vi "Get Distance LUT.vi"() -> (2 "Info":T1, 3 "LUT Out":i32[](array[numeric])=[0, 3, 6, 9, 12])   [LabVIEW 2025]
panel:
  in  "Outputs":T1
  out "Max Distance":i32
  out "Step Size":i32=3
  out "Start Distance":i32
  in  "Distance LUT":i32[](array[numeric])=[6, 9, 12, 15, 18]
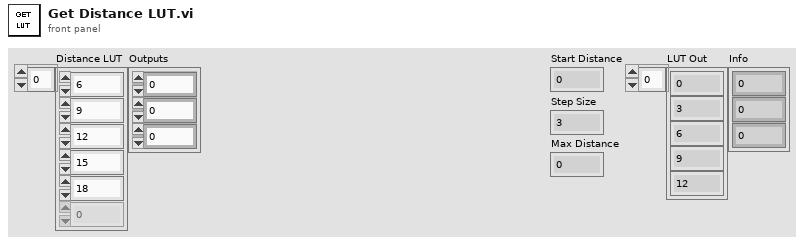
[diagram p1: front panel]
types:
  T1 = cluster{"Start Distance":i32, "Step Size":i32, "Max Distance":i32}
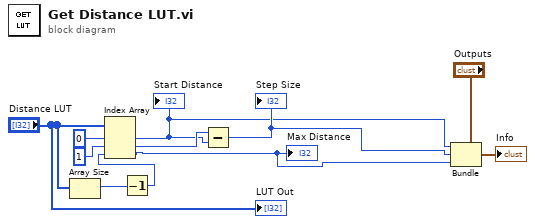
[diagram p0: block diagram]
diagram:
  n1 = Array Size(array="Distance LUT") -> (size(s)=w8:i32)
  n2 = Decrement(x=w8) -> (x-1=w6:i32)
  n3 = Index Array(array="Distance LUT", index #1=0 ("index"), index #2=1 ("index"), index #3=w6) -> (element #1=w3:i32, element #2=w10:i32, element #3=w5:i32)
  "Start Distance" <- w3
  "Max Distance" <- w5
  n4 = Subtract(x=w10, y=w3) -> (x-y=w4:i32)
  "Step Size" <- w4
  n5 = Bundle(cluster="Outputs", "Start Distance"=w3, "Step Size"=w4, "Max Distance"=w5) -> (→"Info":T1)
  "LUT Out" <- "Distance LUT"
